vi "Find Max Pressure.vi"(7 "Error In":errorcluster, 8 "File Path":path, 10 "Pressure":dynamicdata(graph)) -> (0 "Error Out":errorcluster, 1 "File Path Indicator":path, 2 "Interruption Time":dbl, 3 "Pressure":dbl)   [LabVIEW 2013]
uses:
  <vilib>/Waveform/WDTOps.llb/WDT Get XY Value DBL.vi
panel:
  out "Array":dbl[](array[numeric])
  in  "Mark Pressure":bool
  out "Enlarged":dynamicdata(graph)
  out "Pressure":dynamicdata(graph)
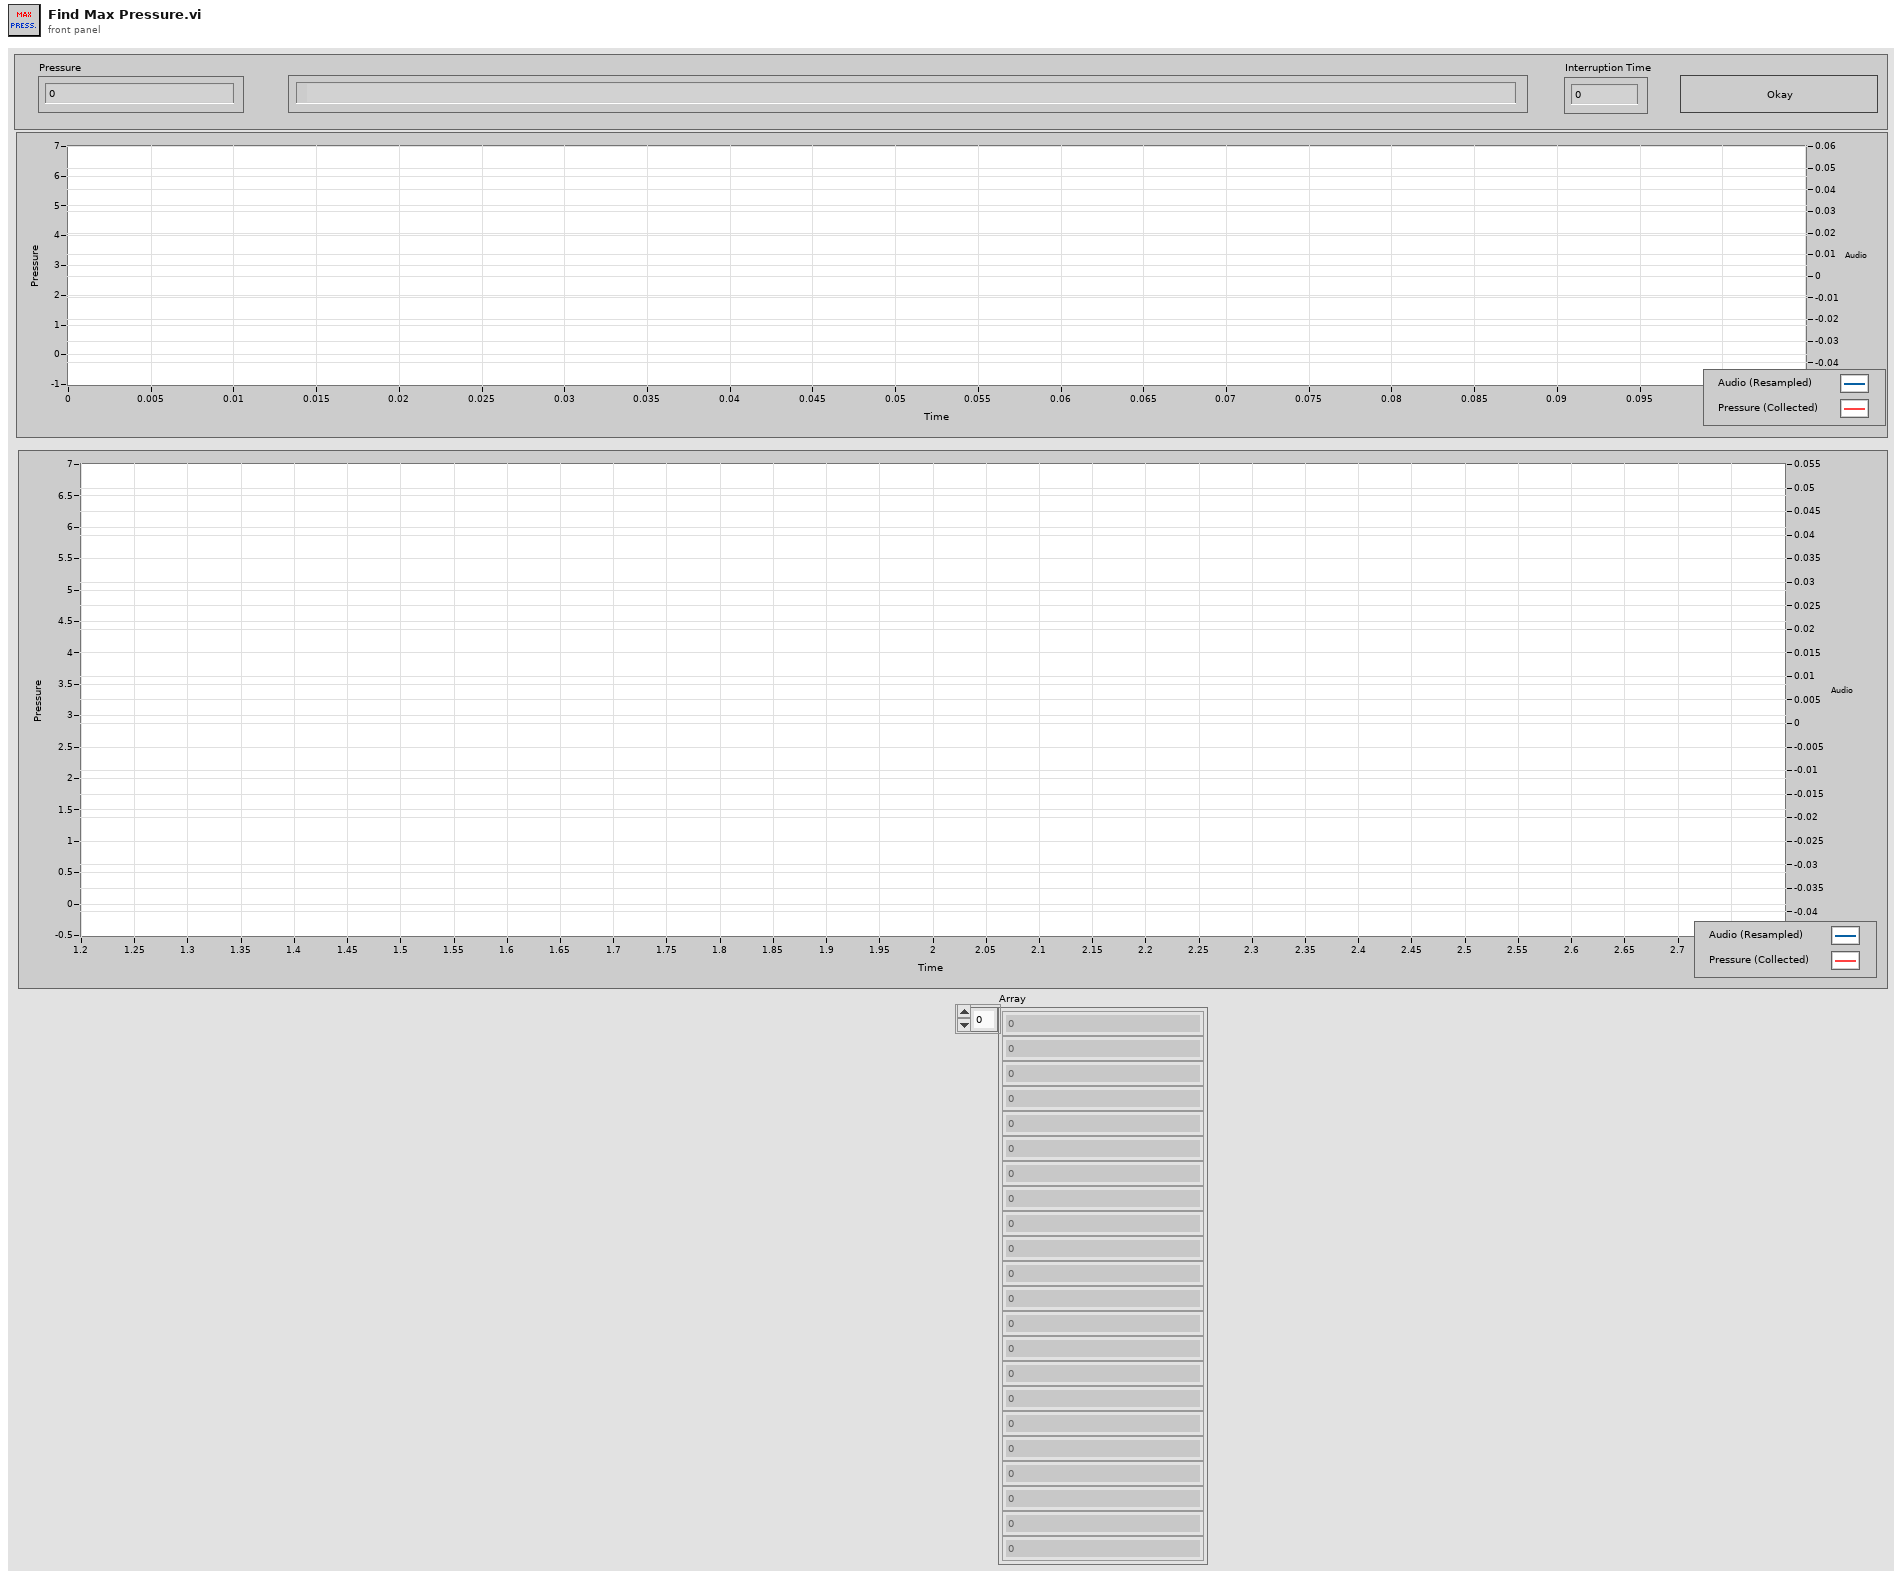
[diagram p1: front panel]
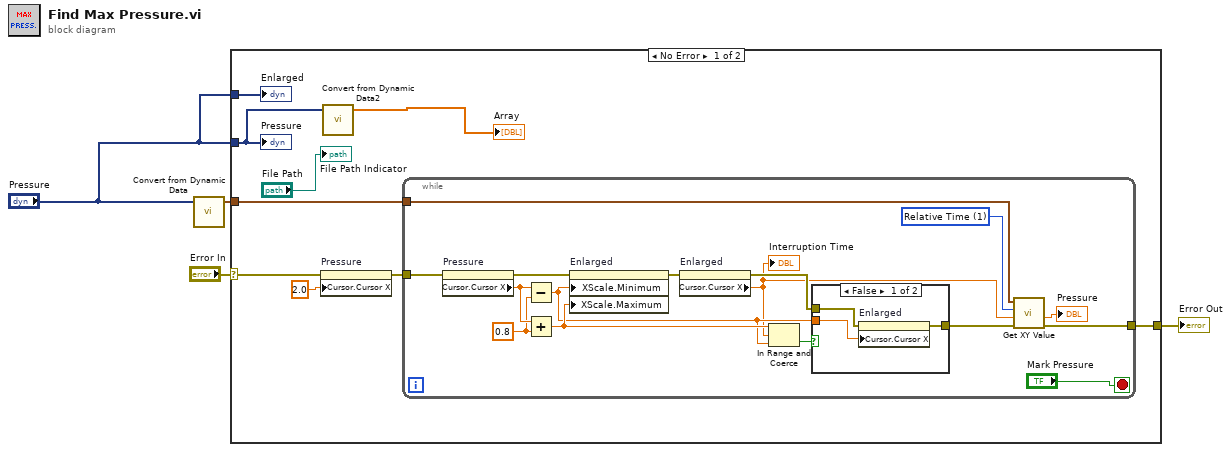
[diagram p0: block diagram]
diagram:
  n1 = call "Convert from Dynamic Data"("Dynamic Data Type"="Pressure") -> ("Waveform"=w2:waveform(dbl))  [unwired: 3 in]
  n2 = case shown="No Error" "Error In" {
    selector: "Error In" -> [w10 w34]
    tunnel: [w12 w34] -> w4
    tunnel: "Pressure" -> [w6 _]
    tunnel: "Pressure" -> [w8 _]
    tunnel: w2 -> [w7 _]
    frame No Error {
      n3 = property on="Pressure" class="WFGraph (strict)"(error in=w10, "Cursor.Cursor X"=2.0 ("Cursor.Cursor Position:Cursor X")) -> (error out=w9:errorcluster)  [unwired: 1 in, 1 out]
      n4 = call "Convert from Dynamic Data2"("Dynamic Data Type"=w6) -> ("Array"=→"Array":dbl[])  [unwired: 3 in]
      n5 = while {
        tunnel: w9 -> [w23]
        tunnel: [w18] -> w12
        tunnel: w7 -> [w16]
        stop <- "Mark Pressure" stop-if-true
        w15 = u16 1 items=["Samples", "Relative Time"] ("Y position format")
        w27 = 0.8 ("y")
        n6 = property on="Pressure" class="WFGraph (strict)"(error in=w23) -> (error out=w22:errorcluster, "Cursor.Cursor X"=w28:dbl)  [unwired: 1 in, 1 out]
        n7 = Subtract(x=w28, y=w27) -> (x-y=w17:dbl)
        n8 = Add(x=w28, y=w27) -> (x+y=w26:dbl)
        n9 = property on="Enlarged" class="WFGraph (strict)"(error in=w22, "XScale.Minimum"=w17, "XScale.Maximum"=w26) -> (error out=w21:errorcluster)  [unwired: 1 in, 1 out]
        n10 = property on="Enlarged" class="WFGraph (strict)"(error in=w21) -> (error out=w20:errorcluster, "Cursor.Cursor X"=w14:dbl)  [unwired: 1 in, 1 out]
        "Interruption Time" <- w14
        n11 = In Range and Coerce(upper limit=w26, x=w14, lower limit=w17) -> (In Range?=w29:bool)  [unwired: 1 out]
        n12 = case shown="False" w29 {
          tunnel: w20 -> [w32 w33]
          tunnel: [w31 w33] -> w19
          tunnel: w17 -> [w30 _]
          frame False {
            n13 = property on="Enlarged" class="WFGraph (strict)"(error in=w32, "Cursor.Cursor X"=w30) -> (error out=w31:errorcluster)  [unwired: 1 in, 1 out]
          }
          frame True {
          }
        }
        n14 = call-poly <vilib>:"Get XY Value.vi"("error in (no error)"=w19, "Y position"=w14, "Y position format"=w15, "waveform in"=w16) -> ("error out"=w18:errorcluster, "Y value"=→"Pressure":dbl)  [unwired: 3 in, 3 out]
      }
      "File Path Indicator" <- "File Path"
      "Enlarged" <- w8
      "Pressure" <- w6
    }
    frame Error {
    }
  }
  "Error Out" <- w4
